vi "Repeat_pos_sorter.vi"(0 "Concatenated Run Messages":string, 1 "Index":i32) -> (2 "Decision":string, 3 "Delete Row":bool, 4 "Error Severity":string)   [LabVIEW 2010]
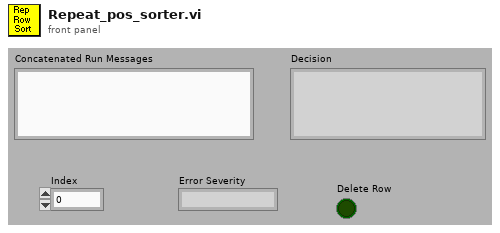
[diagram p1: front panel]
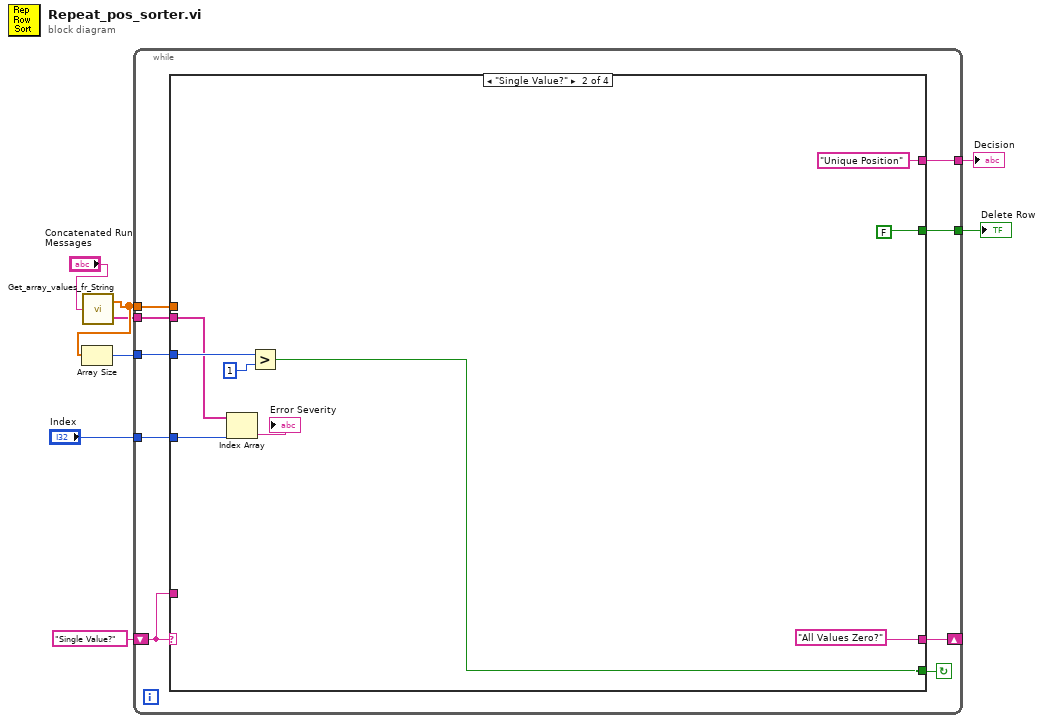
[diagram p0: block diagram]
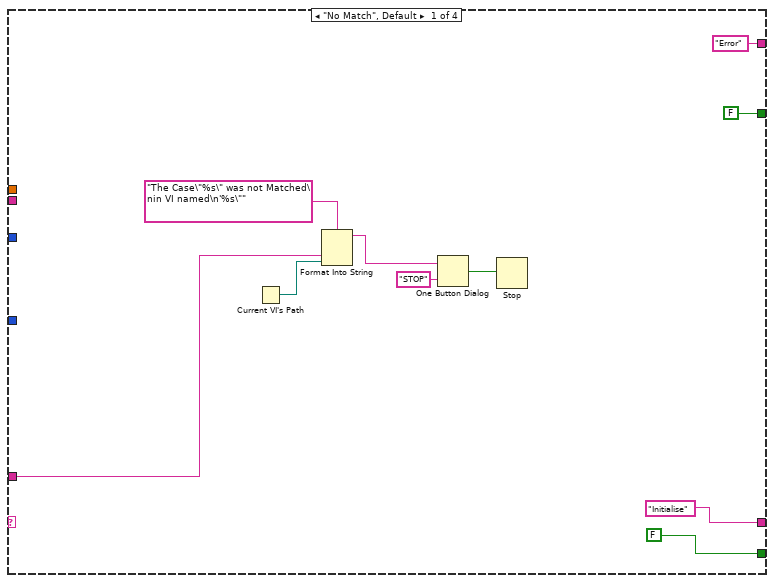
[diagram p2: hidden frame]
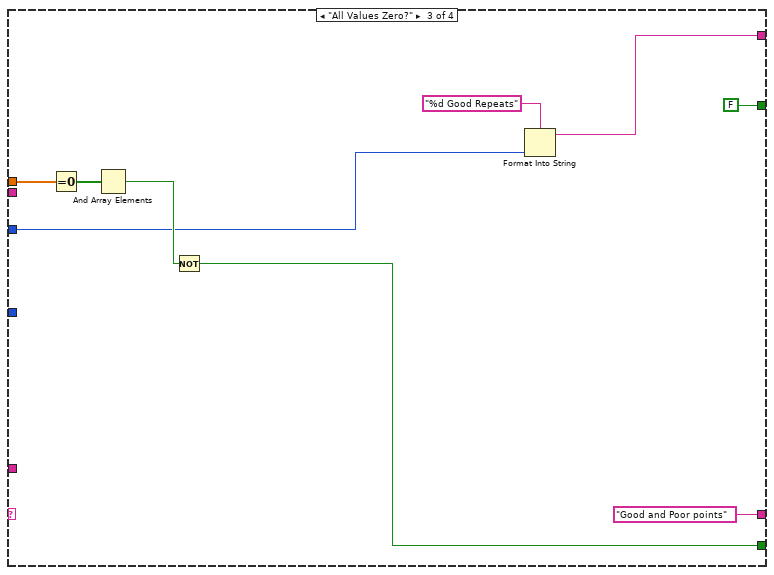
[diagram p3: hidden frame]
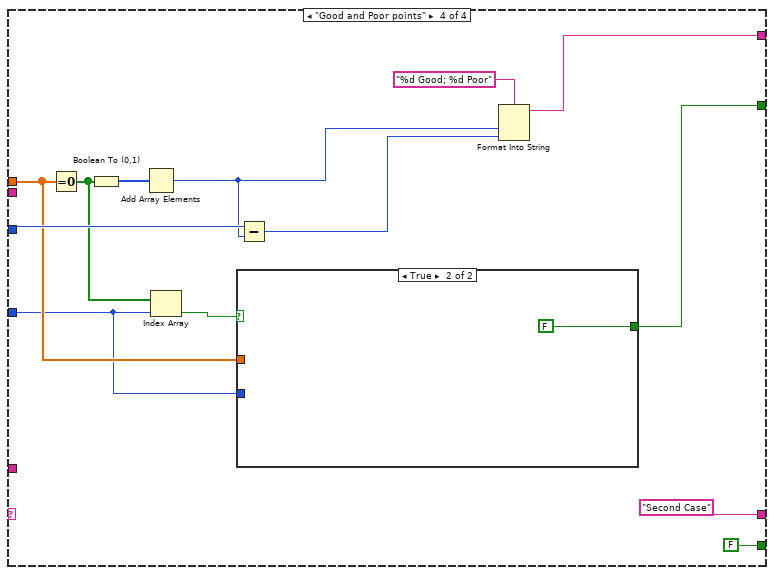
[diagram p4: hidden frame]
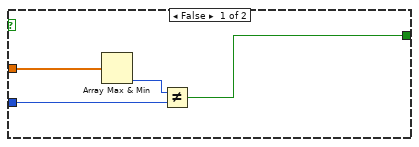
[diagram p5: hidden frame]
diagram:
  n1 = call "Get_array_values_fr_String.vi"("String Value"="Concatenated Run Messages") -> ("Numeric Array"=w4:dbl[], "String array"=w1:string[])
  n2 = Array Size(array=w4) -> (size(s)=w3:i32)
  n3 = while {
    shift-left: "Single Value?" -> [w15]
    shift-right: [w16] -> _
    tunnel: w4 -> [w14]
    tunnel: [w13] -> w6
    tunnel: [w12] -> w5
    tunnel: w3 -> [w11]
    tunnel: "Index" -> [w10]
    tunnel: w1 -> [w9]
    stop <- w17 continue-if-true
    n4 = case shown="\"Single Value?\"" w15 {
      tunnel: [FALSE w34 w41 FALSE] -> w17
      tunnel: ["Initialise" "All Values Zero?" "Good and Poor points" "Second Case"] -> w16
      tunnel: w15 -> [w22 _ _ _]
      tunnel: w14 -> [_ _ w44 w48]
      tunnel: ["Error" "Unique Position" w37 w52] -> w13
      tunnel: [FALSE ("Delete Row") FALSE ("Delete Row") FALSE ("Delete Row") w49] -> w12
      tunnel: w11 -> [_ w31 w39 w55]
      tunnel: w10 -> [_ w29 _ w47]
      tunnel: w9 -> [_ w30 _ _]
      frame "No Match", Default {
        n5 = Current VI's Path() -> (path=w21:path)
        n6 = Format Into String(format string="The Case\"%s\" was not Matched\nin VI named\n'%s\"" ("Format String"), w22, w21) -> (resulting string=w25:string)  [unwired: 2 in, 1 out]
        n7 = One Button Dialog(message=w25, button name ("OK")="STOP") -> (true=w23:bool)
        n8 = Stop(stop? (T)=w23) -> ()
      }
      frame "Single Value?" {
        n9 = Index Array(array=w30, index=w29) -> (element=→"Error Severity":string)
        n10 = Greater?(x=w31, y=1) -> (0:w34:bool)
      }
      frame "All Values Zero?" {
        n11 = Equal To 0?(x=w44) -> (x = 0?=w43:bool[])
        n12 = And Array Elements(Boolean array=w43) -> (logical AND=w42:bool)
        n13 = Not(x=w42) -> (.not. x?=w41:bool)
        n14 = Format Into String(format string="%d Good Repeats", w39) -> (resulting string=w37:string)  [unwired: 2 in, 1 out]
      }
      frame "Good and Poor points" {
        n15 = Equal To 0?(x=w48) -> (x = 0?=w51:bool[])
        n16 = Boolean To (0,1)(Boolean=w51) -> (0, 1=w56:i16[])
        n17 = Add Array Elements(numeric array=w56) -> (sum=w54:i16)
        n18 = Index Array(array=w51, index=w47) -> (element=w50:bool)
        n19 = case shown="True" w50 {
          tunnel: [w59 FALSE] -> w49
          tunnel: w48 -> [w62 _]
          tunnel: w47 -> [w60 _]
          frame False {
            n20 = Array Max & Min(array=w62) -> (min index (indices)=w61:i32)  [unwired: 3 out]
            n21 = Not Equal?(x=w61, y=w60) -> (x != y?=w59:bool)
          }
          frame True {
          }
        }
        n22 = Subtract(x=w55, y=w54) -> (x-y=w53:i32)
        n23 = Format Into String(format string="%d Good; %d Poor", w54, w53) -> (resulting string=w52:string)  [unwired: 2 in, 1 out]
      }
    }
  }
  "Decision" <- w6
  "Delete Row" <- w5
